vi "main.vi"(8 "error in (no error)":errorcluster) -> (0 "error out":errorcluster)   [LabVIEW 2017]
doc: "The main VI of Test Special Program for CANDU project"
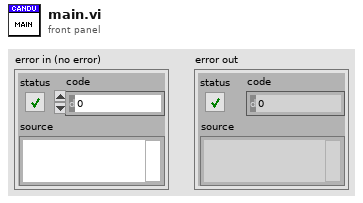
[diagram p1: front panel]
types:
  T1 = typedef "View Model.ctl" = cluster{"Shared Model":T2, "Error Model":T3, "Controller Model":T4, "TDMS Model":T5}
  T2 = typedef "Shared Model.ctl" = cluster{"Stop":refnum<user-event>, "Stop DVR":refnum<data-value>}
  T3 = typedef "Error Model.ctl" = cluster{"Error":refnum<user-event>}
  T4 = typedef "Controller Model.ctl" = cluster{"Command":refnum<user-event>, "Overhead DVR":refnum<data-value>, "DAQ Data DVR":refnum<data-value>}
  T5 = typedef "TDMS Model.ctl" = cluster{"TDMS Event":refnum<user-event>, "TDMS DVR":refnum<data-value>}
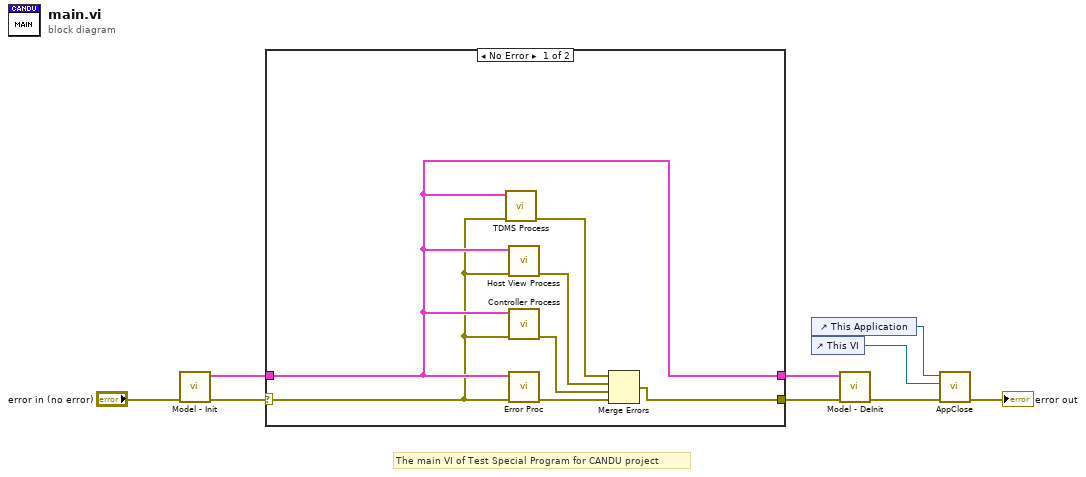
[diagram p0: block diagram]
diagram:
  # "The main VI of Test Special Program for CANDU project"
  n1 = call "Model - Init.vi"("error in (no error)"="error in (no error)") -> ("error out"=w8:errorcluster, "View Model"=w6:T1)  [unwired: 9 in]
  n2 = case shown="No Error" w8 {
    selector: w8 -> [w11 w18]
    tunnel: [w13 w18] -> w7
    tunnel: w6 -> [w12 w17]
    tunnel: [w12 w17] -> w5
    frame No Error {
      n3 = call "TDMS Process.vi"("error in (no error)"=w11, "View Model"=w12) -> ("error out"=w10:errorcluster)  [unwired: 9 in]
      n4 = call "Host View Process.vi"("error in (no error)"=w11, "View Model"=w12) -> ("error out"=w14:errorcluster)  [unwired: 9 in]
      n5 = call "Controller Process.vi"("error in"=w11, "View Model"=w12) -> ("error out"=w15:errorcluster)  [unwired: 9 in]
      n6 = call "Error Proc.vi"("error in (no error)"=w11, "View Model"=w12) -> ("error out"=w16:errorcluster)  [unwired: 9 in]
      n7 = Merge Errors(w10, w14, w15, w16) -> (w13:errorcluster)
    }
    frame Error {
    }
  }
  n8 = control-ref of="This Application"() -> (w1:refnum<vi>)
  n9 = control-ref of="This VI"() -> (w2:refnum<vi>)
  n10 = call "Model - DeInit.vi"("error in (no error)"=w7, "View Model"=w5) -> ("error out"=w4:errorcluster)  [unwired: 9 in]
  n11 = call "AppClose.vi"("Error In"=w4, "This VI"=w2, "This App"=w1) -> ("Error Out"=→"error out":errorcluster)  [unwired: 8 in]
